vi "Main (Binary Search).vi"() -> ()   [LabVIEW 2020]
uses:
  <vilib>/DAQmx/create/channels.llb/DAQmx Create Channel (DO-Digital Output).vi
panel:
  in  "Beginning Tube Number":i32
  in  "End Tube Number":i32
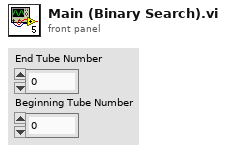
[diagram p1: front panel]
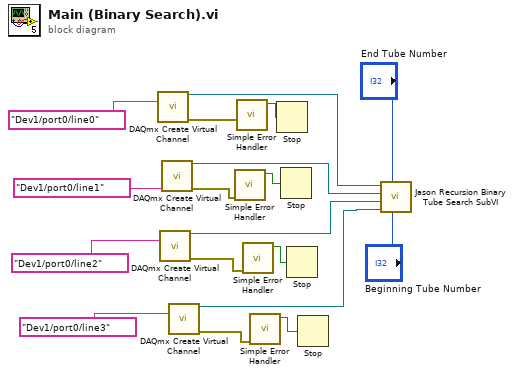
[diagram p0: block diagram]
diagram:
  n1 = call-poly <vilib>:"DAQmx Create Virtual Channel.vi"("lines"=tag "Dev1/port0/line0" ("Data Pin")) -> ("task out"=w6:refnum<k21>, "error out"=w14:errorcluster)  [unwired: 13 in]
  n2 = call-poly <vilib>:"DAQmx Create Virtual Channel.vi"("lines"=tag "Dev1/port0/line2" ("Write Pin")) -> ("task out"=w4:refnum<k21>, "error out"=w12:errorcluster)  [unwired: 13 in]
  n3 = call-poly <vilib>:"DAQmx Create Virtual Channel.vi"("lines"=tag "Dev1/port0/line1" ("Sync Pin")) -> ("task out"=w5:refnum<k21>, "error out"=w13:errorcluster)  [unwired: 13 in]
  n4 = call-poly <vilib>:"DAQmx Create Virtual Channel.vi"("lines"=tag "Dev1/port0/line3" ("Clear Pin")) -> ("task out"=w3:refnum<k21>, "error out"=w11:errorcluster)  [unwired: 13 in]
  n5 = call <vilib>:"Simple Error Handler.vi"("error in (no error)"=w13) -> ("error?"=w7:bool)  [unwired: 4 in, 4 out]
  n6 = call <vilib>:"Simple Error Handler.vi"("error in (no error)"=w14) -> ("error?"=w10:bool)  [unwired: 4 in, 4 out]
  n7 = call <vilib>:"Simple Error Handler.vi"("error in (no error)"=w12) -> ("error?"=w8:bool)  [unwired: 4 in, 4 out]
  n8 = call <vilib>:"Simple Error Handler.vi"("error in (no error)"=w11) -> ("error?"=w9:bool)  [unwired: 4 in, 4 out]
  n9 = Stop(stop? (T)=w10) -> ()
  n10 = Stop(stop? (T)=w7) -> ()
  n11 = Stop(stop? (T)=w8) -> ()
  n12 = Stop(stop? (T)=w9) -> ()
  n13 = call "Jason Recursion Binary Tube Search SubVI.vi"("Beginning Tube Number"="Beginning Tube Number", "End Tube Number"="End Tube Number", "Clear Pin Task In"=w3, "Write Pin Task In"=w4, "Sync Pin Task In"=w5, "Data Pin Task In"=w6) -> ()  [unwired: 2 in, 4 out]
